vi "ErrorHandler.vi"(8 "error in (no error)":errorcluster, 11 "MessageQueue":refnum<queue>) -> (0 "error out":errorcluster, 3 "MessageQueue":refnum<queue>)   [LabVIEW 2018, in "SyncModule.lvlib"]
uses:
  SyncModule.lvlib
  PublicAPI/Arguments/Messages/clMessage.ctl
panel:
  in  "Message (Error)":string="Error"
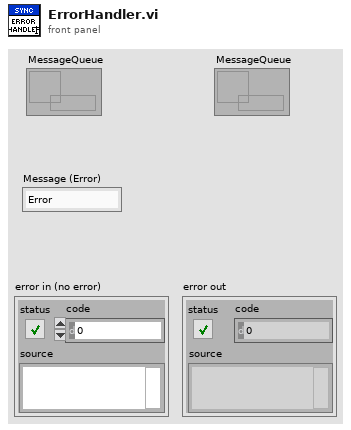
[diagram p1: front panel]
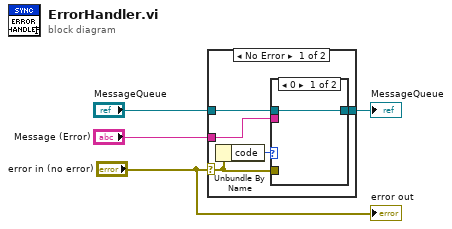
[diagram p0: block diagram]
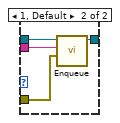
[diagram p2: hidden frame]
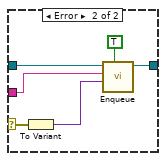
[diagram p3: hidden frame]
diagram:
  n1 = case shown="No Error" "error in (no error)" {
    selector: "error in (no error)" -> [w5 w19]
    tunnel: [w7 w16] -> w2
    tunnel: "MessageQueue" -> [w8 w20]
    tunnel: "Message (Error)" -> [w6 w17]
    frame No Error {
      n2 = Unbundle By Name(w5) -> ("code"=w9:i32)
      n3 = case shown="0" w9 {
        tunnel: w8 -> [w10 w14]
        tunnel: [w10 w13] -> w7
        tunnel: w6 -> [_ w12]
        tunnel: w5 -> [_ w11]
        frame 0 {
        }
        frame 1, Default {
          n4 = call "Enqueue.vi"("Message Data"=w11, "Message"=w12, "MessageQueue"=w14) -> ("MessageQueue"=w13:refnum<queue>)  [unwired: 7 in, 1 out]
        }
      }
    }
    frame Error {
      n5 = To Variant(anything=w19) -> (Variant=w18:variant)
      n6 = call "Enqueue.vi"("Priority (F)"=TRUE, "Message Data"=w18, "Message"=w17, "MessageQueue"=w20) -> ("MessageQueue"=w16:refnum<queue>)  [unwired: 6 in, 1 out]
    }
  }
  "MessageQueue" <- w2
  "error out" <- "error in (no error)"
